vi "Expanded Terminals.vi"(11 "State":T9) -> (3 "Terms":T1)   [LabVIEW 2020, in "Parallel Diagram Block.xnode"]
uses:
  Parallel Diagram Block.xnode
  State.ctl
  Parallel Block/Type Descriptor.ctl
  Parallel Block/Direction.ctl
  Parallel Block/Value Type.ctl
  Parallel Block/Terminal Mode.ctl
  Parallel Block/Terminal Type.ctl
  <vilib>/picture/picture.llb/imagedata.ctl
  <vilib>/XNodeSupport/XNodeTerm4Array.ctl
  <vilib>/XNodeSupport/XNodeTerm4.ctl
  <vilib>/XNodeSupport/XNodeString.ctl
  <vilib>/XNodeSupport/XNodeVariant.ctl
  <vilib>/XNodeSupport/XNodeRect32.ctl
  <vilib>/XNodeSupport/XNodeInt.ctl
  <vilib>/XNodeSupport/XNodeBool.ctl
  <vilib>/XNodeSupport/XNodeTermDirection.ctl
  <vilib>/XNodeSupport/NI_XNodeSupport.lvlib
  Parallel Block/Parallel Block.lvlib
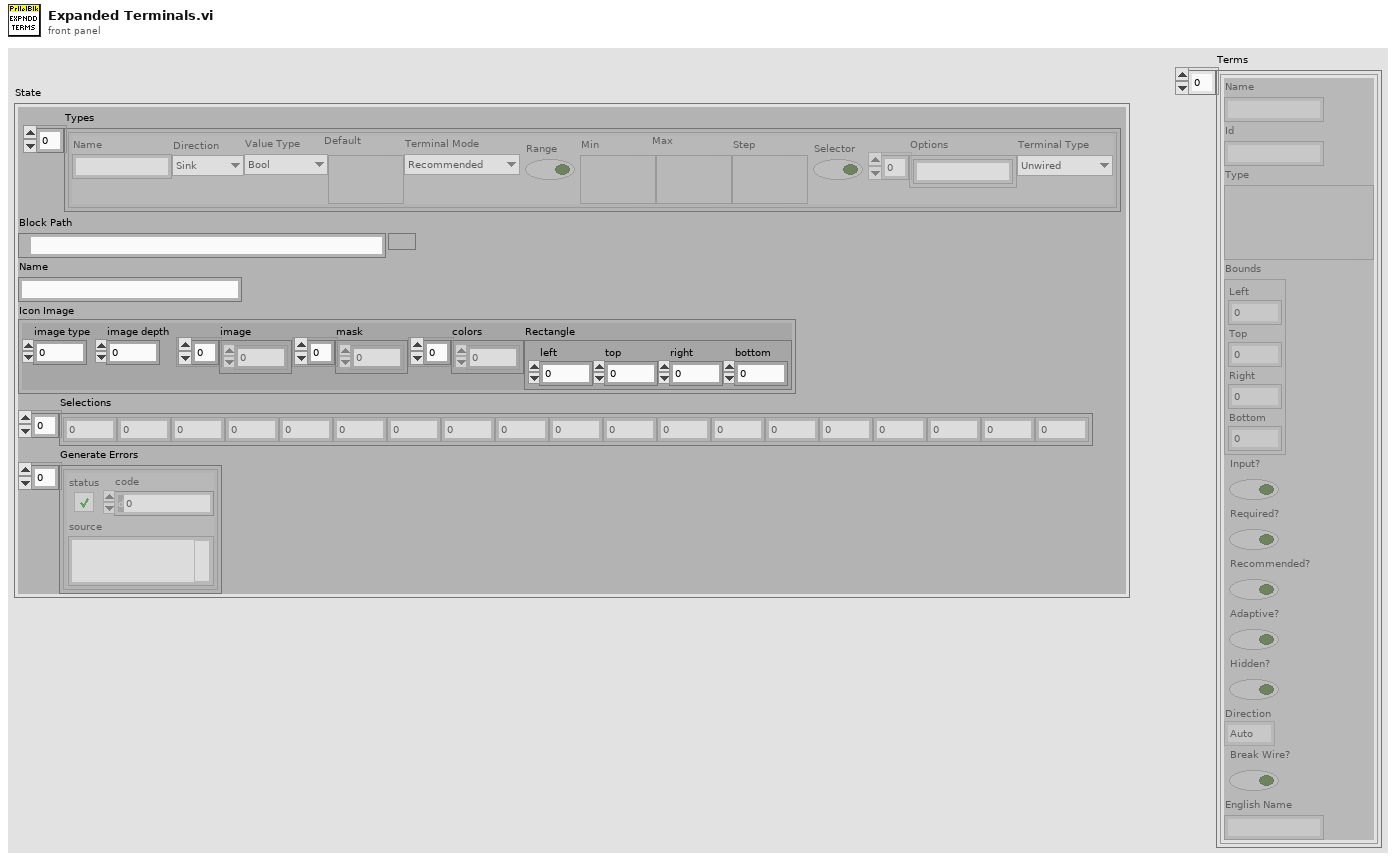
[diagram p1: front panel]
types:
  T1 = typedef "NI_XNodeSupport.lvlib/XNodeTerm4Array.ctl" = T2[]
  T2 = typedef "NI_XNodeSupport.lvlib/XNodeTerm4.ctl" = cluster{"Name":T3, "Id":T3, "Type":T4, "Bounds":T5, "Input?":T7, "Required?":T7, "Recommended?":T7, "Adaptive?":T7, "Hidden?":T7, "Direction":T8, "Break Wire?":T7, "English Name":T3}
  T3 = typedef "NI_XNodeSupport.lvlib/XNodeString.ctl" = string
  T4 = typedef "NI_XNodeSupport.lvlib/XNodeVariant.ctl" = variant
  T5 = typedef "NI_XNodeSupport.lvlib/XNodeRect32.ctl" = cluster{"Left":T6, "Top":T6, "Right":T6, "Bottom":T6}
  T6 = typedef "NI_XNodeSupport.lvlib/XNodeInt.ctl" = i32
  T7 = typedef "NI_XNodeSupport.lvlib/XNodeBool.ctl" = bool
  T8 = typedef "NI_XNodeSupport.lvlib/XNodeTermDirection.ctl" = enum32{"Auto", "Up", "Down", "Left", "Right", "Center"}
  T9 = typedef "Parallel Diagram Block.xnode/State.ctl" = cluster{"Types":T10[], "Block Path":path, "Name":string, "Icon Image":T15, "Selections":i32[], "Generate Errors":errorcluster[]}
  T10 = typedef "Parallel Block.lvlib/Type Descriptor.ctl" = cluster{"Name":string, "Direction":T11, "Value Type":T12, "Default":variant, "Terminal Mode":T13, "Range":bool, "Min":variant, "Max":variant, "Step":variant, "Selector":bool, "Options":string[], "Terminal Type":T14}
  T11 = typedef "Parallel Block.lvlib/Direction.ctl" = enum16{"Sink", "Source"}
  T12 = typedef "Parallel Block.lvlib/Value Type.ctl" = enum16{"Unknown", "Bool", "U8", "U16", "U32", "U64", "I8", "I16", "I32", "I64", "SGL", "DBL", "CSG", "CDB", "CDBWfm", "String", "DBLWfm"}
  T13 = typedef "Parallel Block.lvlib/Terminal Mode.ctl" = enum16{"Recommended", "Required", "None"}
  T14 = typedef "Parallel Block.lvlib/Terminal Type.ctl" = enum16{"Unwired", "BadType", "Connection", "Value", "Control Ref", "BadRefType"}
  T15 = typedef "imagedata.ctl" = cluster{"image type":i32, "image depth":i32, "image":u8[], "mask":u8[], "colors":u32[], "Rectangle":cluster{"left":i16, "top":i16, "right":i16, "bottom":i16}}
  T16 = cluster{"left":i16, "top":i16, "right":i16, "bottom":i16}
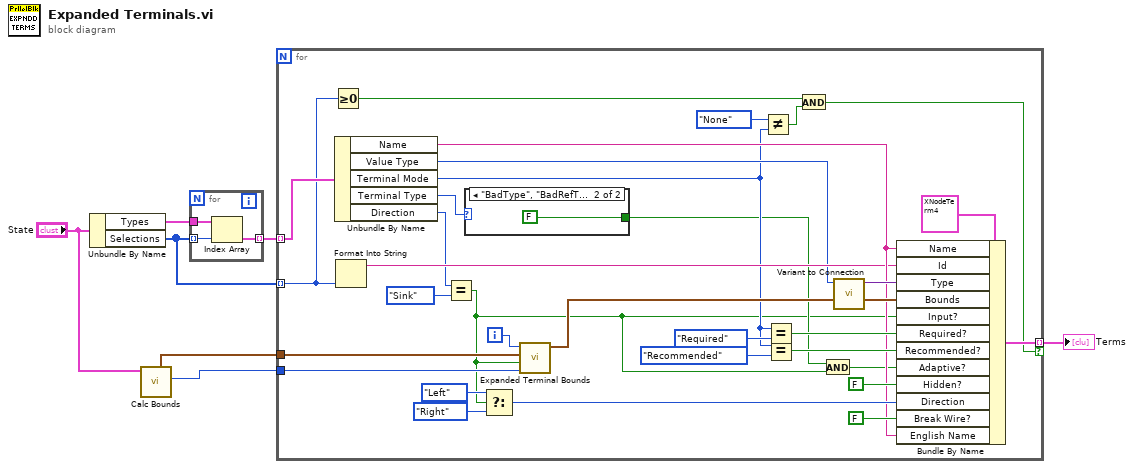
[diagram p0: block diagram]
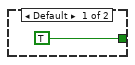
[diagram p2: hidden frame]
diagram:
  n1 = Unbundle By Name("State") -> ("Types"=w3:T10[], "Selections"=w1:i32[])
  n2 = call "Calc Bounds.vi"("State"="State") -> ("Header"=w4:i32, "Bounds Without Terminals"=w6:T16)  [unwired: 6 in, 3 out]
  n3 = for {
    tunnel: w3 -> [w10]
    tunnel: w1 -> [w9] mode=indexing
    tunnel: [w8] -> w2 mode=indexing
    n4 = Index Array(array=w10, index=w9) -> (element=w8:T10)
  }
  n5 = for {
    tunnel: w6 -> [w35]
    tunnel: [w32] -> w5 mode=indexing if=w17
    tunnel: w4 -> [w31]
    tunnel: w2 -> [w25] mode=indexing
    tunnel: w1 -> [w16] mode=indexing
    i -> [w34]
    n6 = Greater Or Equal To 0?(x=w16) -> (x >= 0?=w15:bool)
    n7 = Unbundle By Name(w25) -> ("Name"=w24:string, "Value Type"=w22:T12, "Terminal Mode"=w19:T13, "Terminal Type"=w14:T14, "Direction"=w21:T11)
    n8 = Format Into String(w16) -> (resulting string=w23:string)  [unwired: 3 in, 1 out]
    n9 = Equal?(x=w21, y=Direction."Sink") -> (x = y?=w11:bool)
    n10 = case shown="\"BadType\", \"BadRefType\"" w14 {
      tunnel: [TRUE FALSE] -> w12
      frame Default {
      }
      frame "BadType", "BadRefType" {
      }
    }
    n11 = Select(t=XNodeTermDirection."Left" ("Direction"), s=w11, f=XNodeTermDirection."Right" ("Direction")) -> (s? t:f=w39:T8)
    n12 = call "Expanded Terminal Bounds.vi"("Header"=w31, "Input"=w11, "Border Without Terminals"=w35, "Index"=w34) -> ("Bounds"=w33:T5)  [unwired: 7 in]
    n13 = Not Equal?(x=Terminal_Mode."None", y=w19) -> (x != y?=w18:bool)
    n14 = Equal?(x=w19, y=Terminal_Mode."Required") -> (x = y?=w30:bool)
    n15 = Equal?(x=w19, y=Terminal_Mode."Recommended") -> (x = y?=w29:bool)
    n16 = And(x=w15, y=w18) -> (x .and. y?=w17:bool)
    n17 = And(x=w12, y=w11) -> (x .and. y?=w13:bool)
    n18 = call "Variant to Connection.vi"("Value Type"=w22) -> ("Connection Class"=w36:variant)  [unwired: 10 in]
    n19 = Bundle By Name(cluster=T2 {"Name"="", "Id"="", "Type"=variant, "Bounds"={"Left"=0, "Top"=0, "Right"=0, "Bottom"=0}, "Input?"=FALSE, "Required?"=FALSE, "Recommended?"=FALSE, "Adaptive?"=FALSE, "Hidden?"=FALSE, "Direction"=enum."Auto", "Break Wire?"=FALSE, "English Name"=""} ("Term 4"), "Name"=w24, "Id"=w23, "Type"=w36, "Bounds"=w33, "Input?"=w11, "Required?"=w30, "Recommended?"=w29, "Adaptive?"=w13, "Hidden?"=T7 FALSE, "Direction"=w39, "Break Wire?"=T7 FALSE, "English Name"=w24) -> (w32:T2)
  }
  "Terms" <- w5
